vi "SUB waveform2XY.vi"(1 "waveform":waveform(dbl)) -> (0 "XYWave":cluster{dbl[], dbl[]})   [LabVIEW 2017]
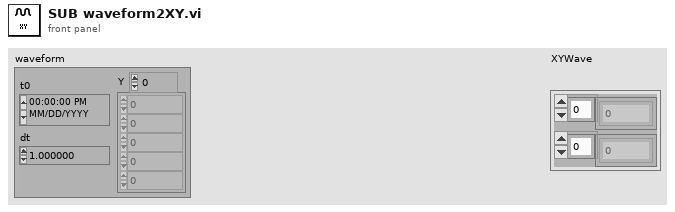
[diagram p1: front panel]
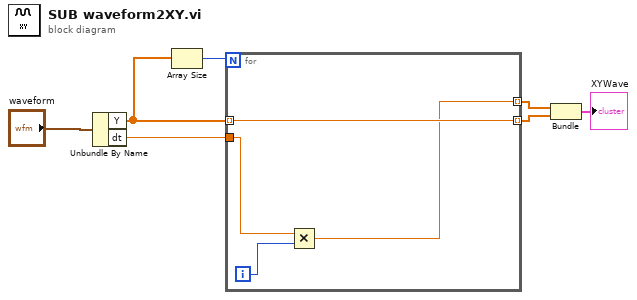
[diagram p0: block diagram]
diagram:
  n1 = Unbundle By Name("waveform") -> ("Y"=w5:dbl[], "dt"=w4:dbl)
  n2 = Array Size(array=w5) -> (size(s)=w6:i32)
  n3 = for {
    N: w6 -> [_]
    tunnel: w5 -> [w11] mode=indexing
    tunnel: [w11] -> w2 mode=indexing
    tunnel: w4 -> [w9]
    tunnel: [w8] -> w3 mode=indexing
    i -> [w10]
    n4 = Multiply(x=w9, y=w10) -> (x*y=w8:dbl)
  }
  n5 = Bundle(w3, w2) -> (→"XYWave":cluster{dbl[], dbl[]})  [unwired: 1 in]
